vi "Insight_Telnet - Proper Close.vi"(2 "error in":errorcluster, 3 "telnet connection":T1) -> (0 "error out":errorcluster)   [LabVIEW 2015]
uses:
  Telnet Session.ctl
panel:
  out "telnet connection out":T1
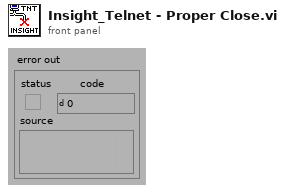
[diagram p1: front panel]
types:
  T1 = typedef "Telnet Session.ctl" = refnum<k1>
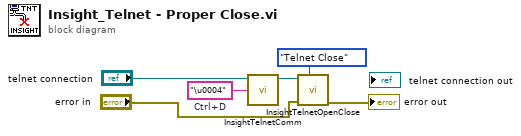
[diagram p0: block diagram]
diagram:
  w6 = "\u0004"  # Ctrl+D
  n1 = call "InsightTelnetComm.vi"("write buffer (\"\")"=w6, "telnet connection"="telnet connection") -> ("telnet  connection out"=w5:T1)  [unwired: 5 in, 2 out]
  n2 = call "InsightTelnetOpenClose.vi"("telnet connection"=w5, "error in (no error)"="error in", "Method"=enum16{"Telnet Open", "Telnet Close"}."Telnet Close") -> ("error out"=→"error out":errorcluster)  [unwired: 6 in, 1 out]
